vi "se_clocks.vi"(6 "haltScan":bool, 7 "se.p.resetClocks":T1, 8 "stepSlow":bool, 9 "stepScan":bool, 10 "moveRates":T5, 11 "se.p.clocks":T2={"outputRate"=50, "fastDecFactor"=0, "outWaveSizeFast"=0, "pplUpsampling"=0, "numLines"=0, "se.p.fastInvDec"=0.0, "se.p.slowUpStep"=0.0, "se.p.outWaveSizeSlow"=0, "blankingMax"=0, "se.p.fastBlanking"={"startFwd"=0, "endFwd"=0, "startBwd"=0, "endBwd"=0, "disableBlanking"=FALSE, "useCoarseCounter"=TRUE}}) -> (0 "moveIndices":cluster{"index":u16, "next":u16}, 1 "indices":T3, 2 "clocks":T4, 3 "fastIndices":T6)   [LabVIEW 2016]
uses:
  <instrlib>/_niInstr/Basic Elements/v1/FPGA/niInstr Basic Elements v1 FPGA.lvlib
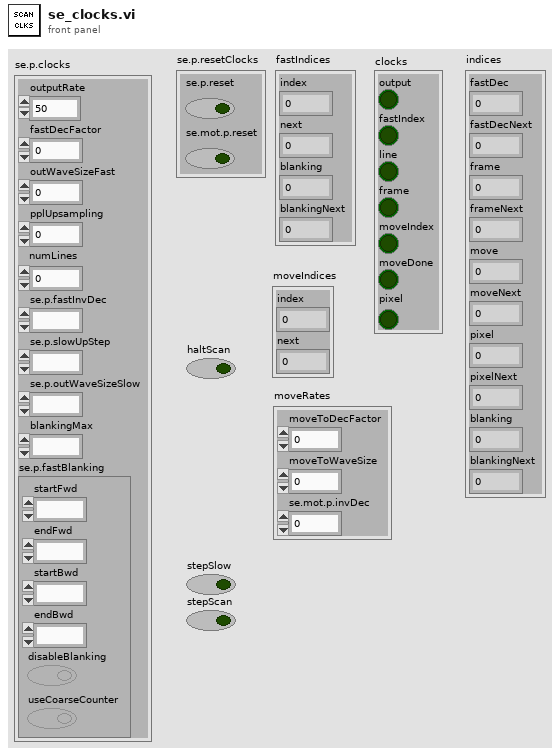
[diagram p1: front panel]
types:
  T1 = cluster{"se.p.reset":bool, "se.mot.p.reset":bool}
  T2 = cluster{"outputRate":u16, "fastDecFactor":u16, "outWaveSizeFast":u16, "pplUpsampling":u16, "numLines":u16, "se.p.fastInvDec":fxp<+,22,0>, "se.p.slowUpStep":fxp<+,22,0>, "se.p.outWaveSizeSlow":u16, "blankingMax":u32, "se.p.fastBlanking":cluster{"startFwd":u32, "endFwd":u32, "startBwd":u32, "endBwd":u32, "disableBlanking":bool, "useCoarseCounter":bool}}
  T3 = cluster{"fastDec":u16, "fastDecNext":u16, "frame":u16, "frameNext":u16, "move":u16, "moveNext":u16, "pixel":u16, "pixelNext":u16, "blanking":u32, "blankingNext":u32}
  T4 = cluster{"output":bool, "fastIndex":bool, "line":bool, "frame":bool, "moveIndex":bool, "moveDone":bool, "pixel":bool}
  T5 = cluster{"moveToDecFactor":u16, "moveToWaveSize":u16, "se.mot.p.invDec":fxp<+,16,0>}
  T6 = cluster{"index":u16, "next":u16, "blanking":u32, "blankingNext":u32}
  T7 = cluster{"index":u16, "next":u16, "index":u32, "next":u32}
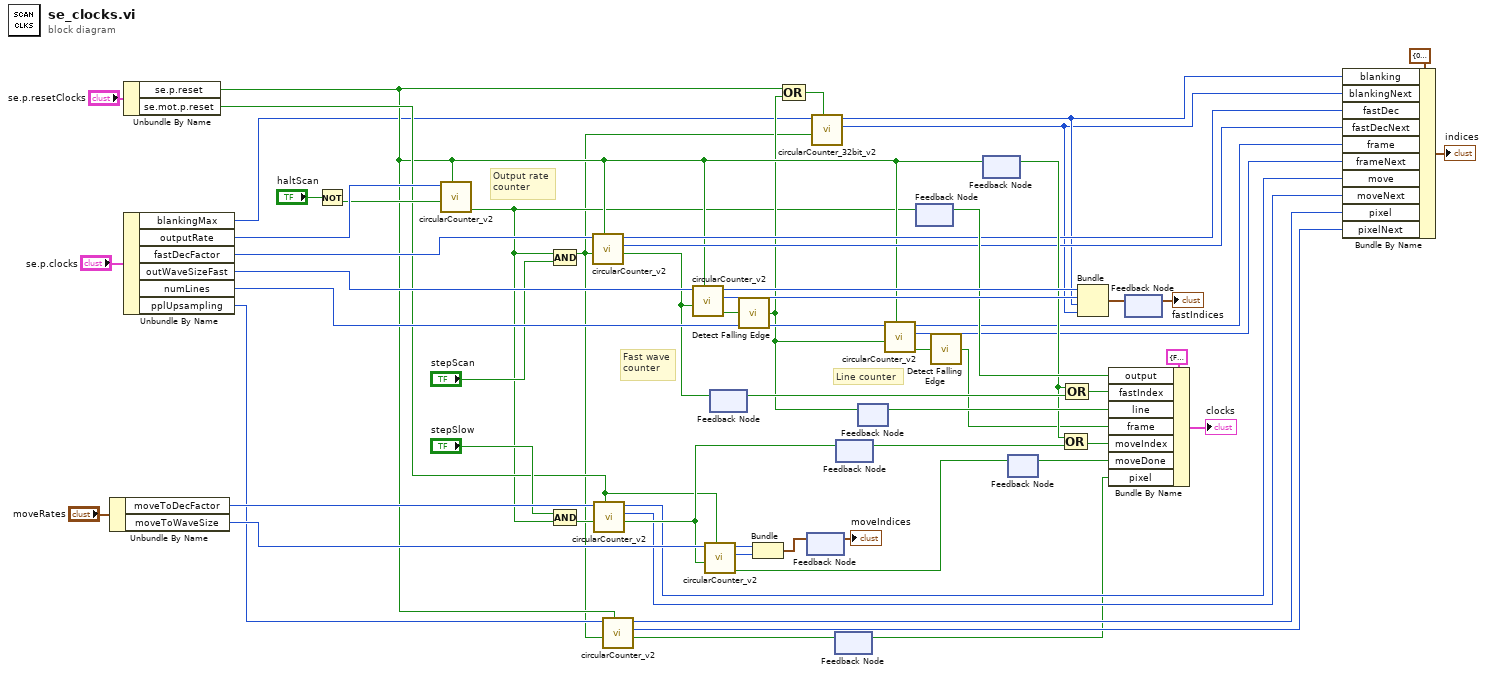
[diagram p0: block diagram]
diagram:
  # "Output rate\ncounter"
  # "Fast wave\ncounter"
  # "Line counter"
  n1 = Unbundle By Name("moveRates") -> ("moveToDecFactor"=w53:u16, "moveToWaveSize"=w52:u16)
  n2 = Unbundle By Name("se.p.resetClocks") -> ("se.p.reset"=w12:bool, "se.mot.p.reset"=w14:bool)
  n3 = Unbundle By Name("se.p.clocks") -> ("blankingMax"=w3:u32, "outputRate"=w60:u16, "fastDecFactor"=w58:u16, "outWaveSizeFast"=w57:u16, "numLines"=w47:u16, "pplUpsampling"=w13:u16)
  n4 = Not(x="haltScan") -> (.not. x?=w17:bool)
  n5 = call "circularCounter_v2.vi"("reset"=w12, "doStep"=w17, "maxCount"=w60) -> ("maxReached"=w4:bool)  [unwired: 5 in, 3 out]
  n6 = Compound Arithmetic op=AND(w4, "stepScan") -> (w1:bool)
  n7 = Compound Arithmetic op=AND("stepSlow", w4) -> (w32:bool)
  n8 = call "circularCounter_v2.vi"("reset"=w12, "doStep"=w1, "maxCount"=w58) -> ("maxPulse"=w20:bool, "next"=w29:u16, "index"=w30:u16)  [unwired: 5 in, 1 out]
  n9 = call "circularCounter_v2.vi"("reset"=w14, "doStep"=w32, "maxCount"=w53) -> ("maxPulse"=w33:bool, "next"=w25:u16, "index"=w26:u16)  [unwired: 5 in, 1 out]
  n10 = call "circularCounter_v2.vi"("reset"=w12, "doStep"=w1, "maxCount"=w13) -> ("maxPulse"=w2:bool, "next"=w23:u16, "index"=w24:u16)  [unwired: 5 in, 1 out]
  n11 = call "circularCounter_v2.vi"("reset"=w12, "doStep"=w20, "maxCount"=w57) -> ("maxReached"=w46:bool, "next"=w55:u16, "index"=w56:u16)  [unwired: 5 in, 1 out]
  n12 = call "circularCounter_v2.vi"("reset"=w14, "doStep"=w33, "maxCount"=w52) -> ("maxReached"=w48:bool, "next"=w50:u16, "index"=w51:u16)  [unwired: 5 in, 1 out]
  n13 = feedback-in #1(w20) -> ()
  n14 = feedback #1() -> (w39:bool)  [unwired: 1 in]
  n15 = call <instrlib>:"Detect Falling Edge.vi"("signal"=w46) -> ("edge detected"=w9:bool)  [unwired: 14 in]
  n16 = Bundle("index"=w51, "next"=w50) -> (w49:cluster{"index":u16, "next":u16})  [unwired: 1 in]
  n17 = Compound Arithmetic op=OR(w12, w9) -> (w10:bool)
  n18 = feedback-in #2(w49) -> ()
  n19 = feedback #2() -> (→"moveIndices":cluster{"index":u16, "next":u16})  [unwired: 1 in]
  n20 = call "circularCounter_32bit_v2.vi"("reset"=w10, "doStep"=w1, "maxCount"=w3) -> ("next"=w5:u32, "index"=w6:u32)  [unwired: 5 in, 2 out]
  n21 = feedback-in #3(w2) -> ()
  n22 = feedback #3() -> (w19:bool)  [unwired: 1 in]
  n23 = feedback-in #4(w33) -> ()
  n24 = feedback #4() -> (w44:bool)  [unwired: 1 in]
  n25 = feedback-in #5(w9) -> ()
  n26 = feedback #5() -> (w45:bool)  [unwired: 1 in]
  n27 = call "circularCounter_v2.vi"("reset"=w12, "doStep"=w9, "maxCount"=w47) -> ("maxReached"=w22:bool, "next"=w27:u16, "index"=w28:u16)  [unwired: 5 in, 1 out]
  n28 = feedback-in #6(w4) -> ()
  n29 = feedback #6() -> (w40:bool)  [unwired: 1 in]
  n30 = call <instrlib>:"Detect Falling Edge.vi"("signal"=w22) -> ("edge detected"=w21:bool)  [unwired: 14 in]
  n31 = feedback-in #7(w12) -> ()
  n32 = feedback #7() -> (w36:bool)  [unwired: 1 in]
  n33 = feedback-in #8(w48) -> ()
  n34 = feedback #8() -> (w43:bool)  [unwired: 1 in]
  n35 = Compound Arithmetic op=OR(w36, w44) -> (w37:bool)
  n36 = Compound Arithmetic op=OR(w36, w39) -> (w38:bool)
  n37 = Bundle("index"=w56, "next"=w55, "index"=w6, "next"=w5) -> (w54:T7)  [unwired: 1 in]
  n38 = Bundle By Name(cluster=T4 {"output"=FALSE, "fastIndex"=FALSE, "line"=FALSE, "frame"=FALSE, "moveIndex"=FALSE, "moveDone"=FALSE, "pixel"=FALSE} ("output cluster"), "output"=w40, "fastIndex"=w38, "line"=w45, "frame"=w21, "moveIndex"=w37, "moveDone"=w43, "pixel"=w19) -> (→"clocks":T4)
  n39 = feedback-in #9(w54) -> ()
  n40 = feedback #9() -> (→"fastIndices":T7)  [unwired: 1 in]
  n41 = Bundle By Name(cluster=T3 {"fastDec"=0, "fastDecNext"=0, "frame"=0, "frameNext"=0, "move"=0, "moveNext"=0, "pixel"=0, "pixelNext"=0, "blanking"=0, "blankingNext"=0} ("indices"), "blanking"=w6, "blankingNext"=w5, "fastDec"=w30, "fastDecNext"=w29, "frame"=w28, "frameNext"=w27, "move"=w26, "moveNext"=w25, "pixel"=w24, "pixelNext"=w23) -> (→"indices":T3)
